vi "Agilent SNA SWP Format Model String.vi"(1 "Model String":string) -> (0 "Model":T1)   [LabVIEW 2011]
uses:
  TypeDefs/Agilent SNA SWP Model.ctl
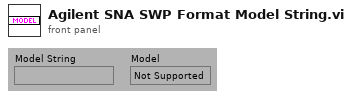
[diagram p1: front panel]
types:
  T1 = typedef "Agilent SNA SWP Model.ctl" = enum16{"Not Supported", "836XXX", "8375XX", "E82X7D"}
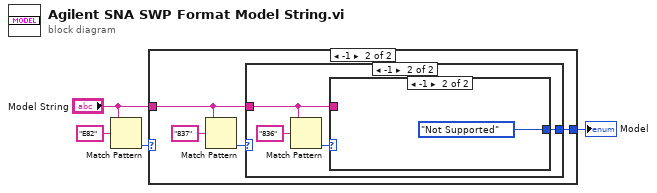
[diagram p0: block diagram]
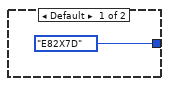
[diagram p2: hidden frame]
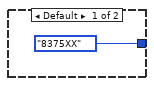
[diagram p3: hidden frame]
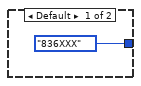
[diagram p4: hidden frame]
diagram:
  n1 = Match Pattern(string="Model String", regular expression="E82") -> (offset past match=w1:i32)  [unwired: 4 out]
  n2 = case shown="-1" w1 {
    tunnel: [Agilent_SNA_SWP_Model."E82X7D" ("Model") w9] -> w4
    tunnel: "Model String" -> [_ w6]
    frame Default {
    }
    frame -1 {
      n3 = Match Pattern(string=w6, regular expression="837") -> (offset past match=w7:i32)  [unwired: 4 out]
      n4 = case shown="-1" w7 {
        tunnel: w6 -> [_ w11]
        tunnel: [Agilent_SNA_SWP_Model."8375XX" ("Model") w14] -> w9
        frame Default {
        }
        frame -1 {
          n5 = Match Pattern(string=w11, regular expression="836") -> (offset past match=w12:i32)  [unwired: 4 out]
          n6 = case shown="-1" w12 {
            tunnel: [Agilent_SNA_SWP_Model."836XXX" ("Model") Agilent_SNA_SWP_Model."Not Supported" ("Model")] -> w14
            tunnel: w11 -> [_ _]
            frame Default {
            }
            frame -1 {
            }
          }
        }
      }
    }
  }
  "Model" <- w4
